vi "被收处理.vi"(0 "时间":string, 1 "报文":string) -> (14 "结果":string[](array[string]), 18 "校验信息":cluster{"可用？":bool, "功能码":u8, "无crc报文":u8[]})   [LabVIEW 2019]
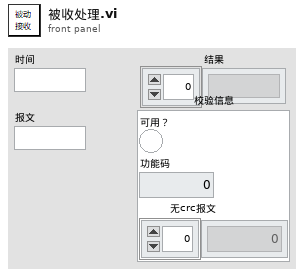
[diagram p1: front panel]
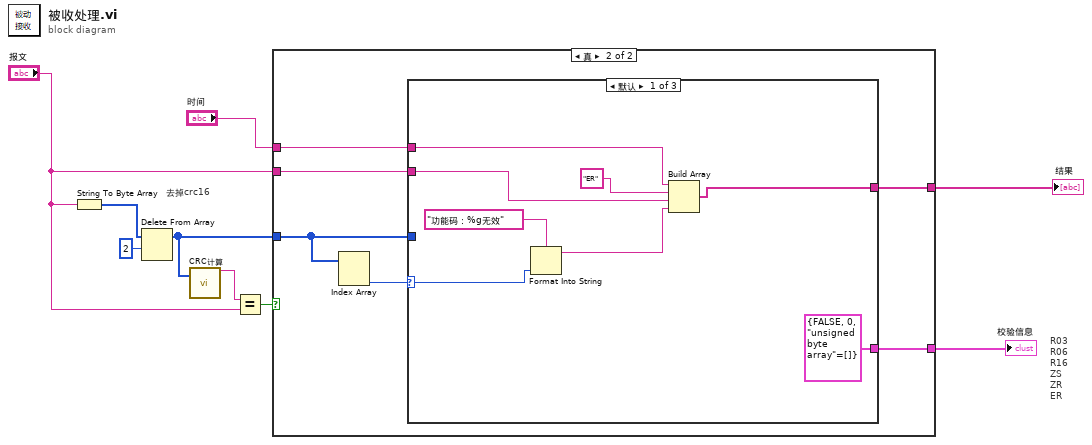
[diagram p0: block diagram]
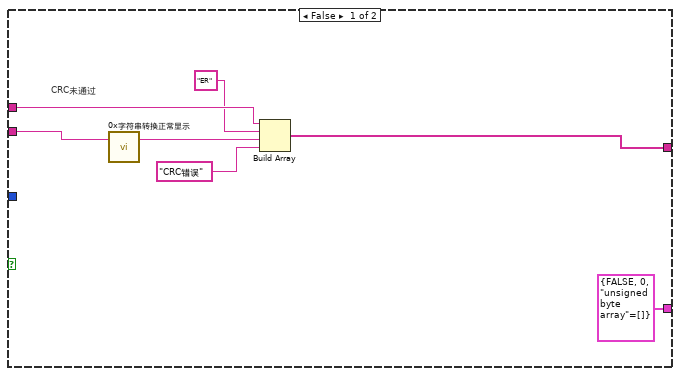
[diagram p2: hidden frame]
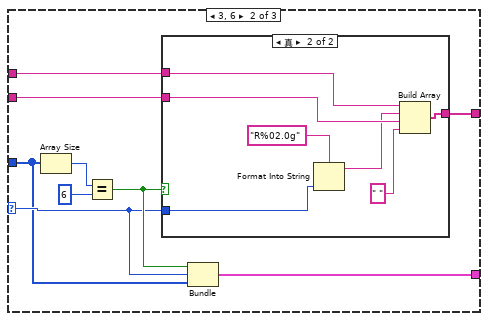
[diagram p3: hidden frame]
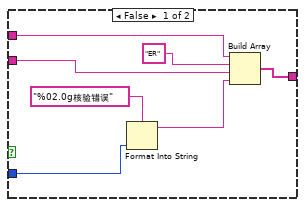
[diagram p4: hidden frame]
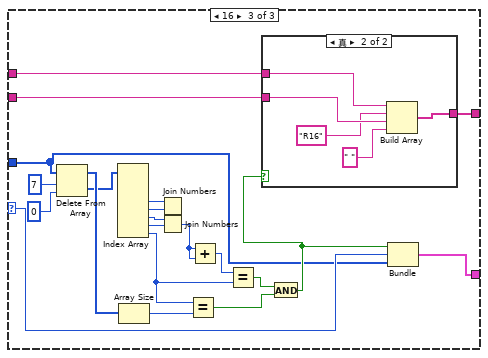
[diagram p5: hidden frame]
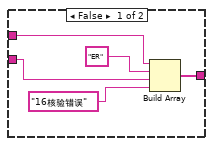
[diagram p6: hidden frame]
diagram:
  # "去掉crc16"
  # "R03\nR06\nR16\nZS\nZR\nER"
  n1 = String To Byte Array(string="报文") -> (unsigned byte array=w9:u8[])
  n2 = Delete From Array(array=w9, length=2 ("长度")) -> (array with subset deleted=w4:u8[])  [unwired: 1 in, 1 out]
  n3 = call "CRC计算.vi"("无校验U8数组"=w4) -> ("计算后字符串"=w7:string)  [unwired: 17 in, 1 out]
  n4 = Equal?(x=w7, y="报文") -> (x = y?=w6:bool)
  n5 = case shown="真" w6 {
    tunnel: [w16 w20] -> w5
    tunnel: "报文" -> [w15 w21]
    tunnel: w4 -> [_ w19]
    tunnel: [cluster{bool, u8, "unsigned byte array":u8[]} {FALSE, 0, "unsigned byte array"=[]} w18] -> w2
    tunnel: "时间" -> [w13 w17]
    frame False {
      # "CRC未通过"
      n6 = call "0x字符串转换正常显示.vi"("普通字符串"=w15) -> ("0x普通字符串"=w12:string)  [unwired: 18 in]
      n7 = Build Array(w13, "ER" ("元素"), w12, "CRC错误" ("元素")) -> (w16:string[])
    }
    frame True {
      n8 = Index Array(array=w19) -> (element #2=w22:u8)  [unwired: 2 in, 1 out]
      n9 = case shown="默认" w22 {
        selector: w22 -> [w30 w33 w56]
        tunnel: w21 -> [w26 w38 w59]
        tunnel: [w27 w35 w58] -> w20
        tunnel: w17 -> [w25 w39 w60]
        tunnel: w19 -> [_ w32 w55]
        tunnel: [cluster{bool, u8, "unsigned byte array":u8[]} {FALSE, 0, "unsigned byte array"=[]} w31 w54] -> w18
        frame Default {
          n10 = Format Into String(format string="功能码：%g无效" ("格式字符串"), w30) -> (resulting string=w28:string)  [unwired: 2 in, 1 out]
          n11 = Build Array(w25, "ER" ("元素"), w26, w28) -> (w27:string[])
        }
        frame 3, 6 {
          n12 = Array Size(array=w32) -> (size(s)=w37:i32)
          n13 = Equal?(x=w37, y=6) -> (x = y?=w34:bool)
          n14 = case shown="真" w34 {
            tunnel: w39 -> [w41 w53]
            tunnel: w38 -> [w42 w52]
            tunnel: [w46 w51] -> w35
            tunnel: w33 -> [w44 w50]
            frame False {
              n15 = Format Into String(format string="%02.0g核验错误" ("元素"), w44) -> (resulting string=w43:string)  [unwired: 2 in, 1 out]
              n16 = Build Array(w41, "ER" ("元素"), w42, w43) -> (w46:string[])
            }
            frame True {
              n17 = Format Into String(format string="R%02.0g" ("格式字符串"), w50) -> (resulting string=w48:string)  [unwired: 2 in, 1 out]
              n18 = Build Array(w53, w48, w52, " " ("元素")) -> (w51:string[])
            }
          }
          n19 = Bundle(w34, w33, "unsigned byte array"=w32) -> (w31:cluster{bool, u8, "unsigned byte array":u8[]})  [unwired: 1 in]
        }
        frame 16 {
          n20 = Delete From Array(array=w55, length=7 ("长度"), index=0 ("索引")) -> (deleted portion=w73:u8[], array with subset deleted=w74:u8[])
          n21 = Index Array(array=w73) -> (element #3=w70:u8, element #4=w71:u8, element #5=w63:u8, element #6=w64:u8, element #7=w67:u8)  [unwired: 7 in, 2 out]
          n22 = Array Size(array=w74) -> (size(s)=w65:i32)
          n23 = Join Numbers(hi=w70, lo=w71) -> ()  [unwired: 1 out]
          n24 = Join Numbers(hi=w63, lo=w64) -> ((hi.lo)=w72:u16)
          n25 = Equal?(x=w67, y=w65) -> (x = y?=w69:bool)
          n26 = Add(x=w72, y=w72) -> (x+y=w66:u16)
          n27 = Equal?(x=w66, y=w67) -> (x = y?=w68:bool)
          n28 = And(x=w68, y=w69) -> (x .and. y?=w57:bool)
          n29 = case shown="真" w57 {
            tunnel: w60 -> [w78 w84]
            tunnel: w59 -> [w77 w83]
            tunnel: [w79 w82] -> w58
            frame False {
              n30 = Build Array(w78, "ER" ("元素"), w77, "16核验错误" ("元素")) -> (w79:string[])
            }
            frame True {
              n31 = Build Array(w84, "R16" ("格式字符串"), w83, " " ("元素")) -> (w82:string[])
            }
          }
          n32 = Bundle(w57, w56, "unsigned byte array"=w55) -> (w54:cluster{bool, u8, "unsigned byte array":u8[]})  [unwired: 1 in]
        }
      }
    }
  }
  "结果" <- w5
  "校验信息" <- w2
